vi "ROI entry-Previous ROI compat-FOV.vi"(8 "error in (no error)":errorcluster, 9 "Proceed":bool=TRUE, 11 "Old ROI file path":path) -> (0 "error out":errorcluster, 1 "Proceed":bool, 3 "Old ROI file path (dup)":path)   [LabVIEW 2017]
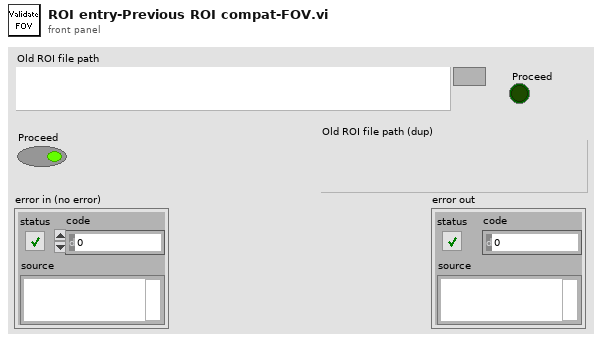
[diagram p1: front panel]
types:
  T1 = typedef "Fixed strings.ctl" = cluster{"ROI file name":string, "Normalised ROI file name":string, "Zplane Pockels values file name":string, "Functional data folder name":string, "Experiment Header file name":string, "Z-stack images folder name":string, "Groups setup rel. path":string, "Groups text file rel. path":string, "TDMS files folder name (F.img)":string, "TDMS files folder name (V.acq)":string, "TDMS files folder name (Pl.acq)":string, "Cycle rel times sequence file":string, "Dynamically called VIs folder name":string, "Time Series folder base name":string}
  T2 = typedef "AOL_Globals.ctl" = cluster{"Imaging Protocol":T3, "Number of POI":u16, "Number of Miniscans":u16, "Number of Trials":u16, "Number of Cycles ":u64, "# Averaged Frames":u16, "Laser power (%)":u8, "Pockels":dbl, "Acquisition Length (sec)":dbl, "Fill time (us)":dbl, "POI Dwell time (us)":dbl, "Miniscan Dwell time per pixel (us)":dbl, "PMT 1":dbl, "PMT 2":dbl, "Back Apperture":dbl, "Frame Size":T4, "Center Frequency":dbl, "Field of View (norm)":dbl, "DwellTime (us)":dbl, "Wavelength (nm)":dbl, "Zoom":dbl, "AOL Z":dbl, "AOL Mode":T5, "GridXY":dbl, "GridZ":dbl, "TriggerPeriod (sec)":dbl, "Number of Pixels in Miniscan":u16, "Experiment folder path":path, "X centre":dbl, "Y centre":dbl, "Angle (degrees)":dbl, "Plane Mode":T6, "Threshold":u16[], "Regenerate Chirps":bool, "Rectangle ROI length (pixels)":u16, "Rectangle ROI height (pixels)":u16, "AOD fill":u16, "StartupDelay":i32, "Samples Wait after Trigger":u16, "Slip Cycle":u32, "Add Cycle":bool, "Functional Mode":T7, "Z Start":dbl, "Z Stop":dbl, "# Planes":i32}
  T3 = typedef "Imaging Protocols enum.ctl" = enum16{"AOL Z-Stack", "Motor Z Stack", "Functional Acquisition", "Single Plane Acquisition", "Volume Acquisition", "Live Imaging", "Live Plane Imaging", "Live Volume Imaging"}
  T4 = typedef "Frame Size.ctl" = u16
  T5 = typedef "AOL modes.ctl" = enum16{"Raster", "Structural", "Pointing", "Mini Scan", "Alignment"}
  T6 = typedef "Plane Mode.ctl" = u16
  T7 = typedef "Functional Mode.ctl" = enum16{"Point", "Line", "Patch", "Plane", "Volume"}
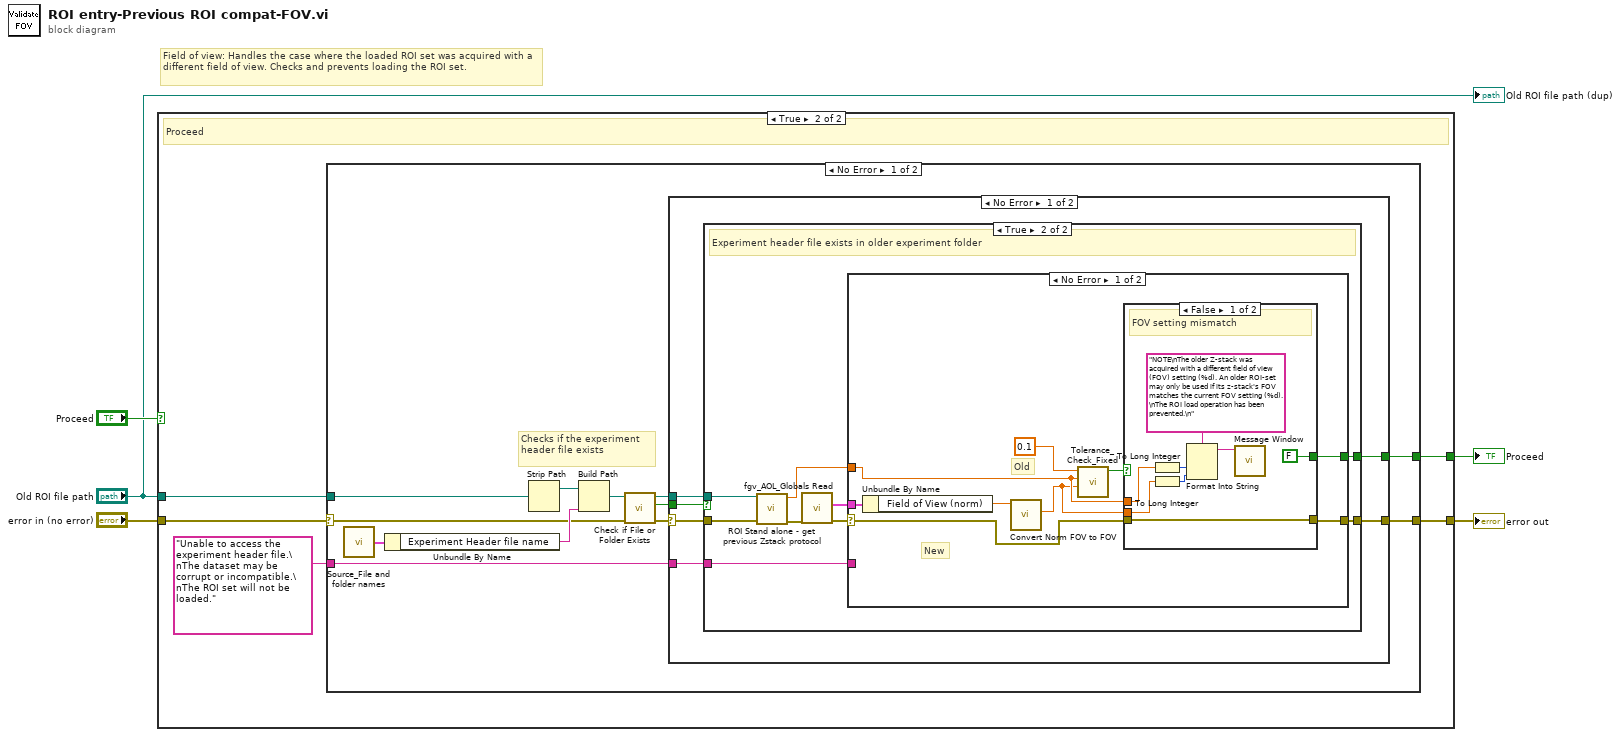
[diagram p0: block diagram]
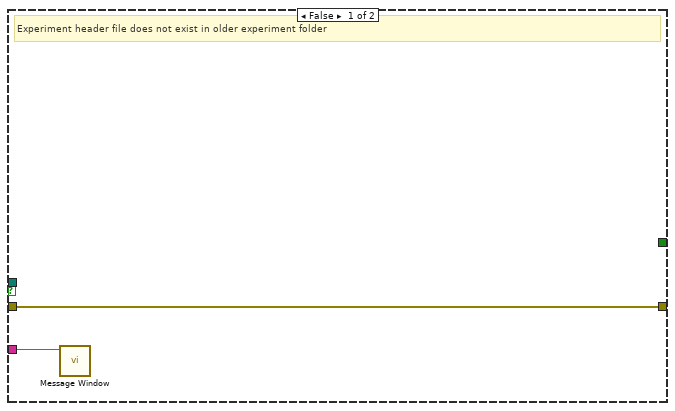
[diagram p3: hidden frame]
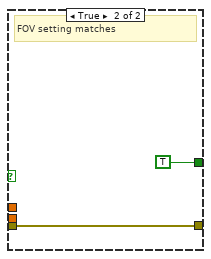
[diagram p4: hidden frame]
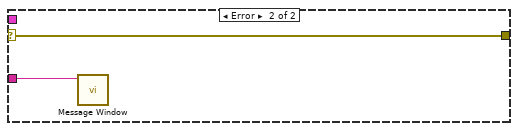
[diagram p5: hidden frame]
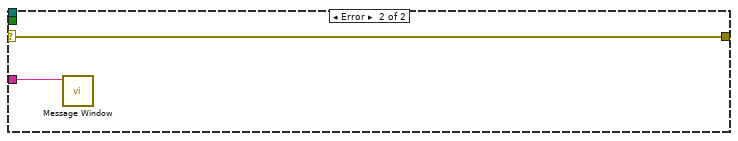
[diagram p6: hidden frame]
diagram:
  # "Field of view: Handles the case where the loaded ROI set was acquired with a different field of view. Checks and prevents loading the ROI set."
  n1 = case shown="True" "Proceed" {
    tunnel: "Old ROI file path" -> [_ w11]
    tunnel: [w6 w9] -> w5
    tunnel: "error in (no error)" -> [w6 w8]
    tunnel: [_ w7] -> w3
    frame False {
      # "Skip"
    }
    frame True {
      # "Proceed"
      n2 = case shown="No Error" w8 {
        selector: w8 -> [w14 w64]
        tunnel: w11 -> [w21 _]
        tunnel: [w17 _] -> w7
        tunnel: [w13 w64] -> w9
        tunnel: "Unable to access the experiment header file.\nThe dataset may be corrupt or incompatible.\nThe ROI set will not be loaded." ("Message string") -> [w12 _]
        frame No Error {
          # "Checks if the experiment header file exists"
          n3 = call "Source_File and folder names.vi"() -> ("Fixed strings"=w22:T1)  [unwired: 1 in]
          n4 = Unbundle By Name(w22) -> ("Experiment Header file name"=w19:string)
          n5 = Strip Path(path=w21) -> (stripped path=w20:path)  [unwired: 1 out]
          n6 = Build Path(base path=w20, name or relative path=w19) -> (appended path=w23:path)
          n7 = call <vilib>:"Check if File or Folder Exists.vi"("error in (no error)"=w14, "path"=w23) -> ("error out"=w15:errorcluster, "file or folder exists?"=w18:bool, "dup path"=w16:path)  [unwired: 7 in]
          n8 = case shown="No Error" w15 {
            selector: w15 -> [w26 w63]
            tunnel: w18 -> [w29 _]
            tunnel: [w28 _] -> w17
            tunnel: w16 -> [w27 _]
            tunnel: [w25 w63] -> w13
            tunnel: w12 -> [w24 w62]
            frame No Error {
              n9 = case shown="True" w29 {
                tunnel: [_ w39] -> w28
                tunnel: w27 -> [_ w34]
                tunnel: w26 -> [w31 w35]
                tunnel: [w31 w38] -> w25
                tunnel: w24 -> [w30 w36]
                frame False {
                  # "Experiment header file does not exist in older experiment folder"
                  n10 = call "Message Window.vi"("Message string"=w30) -> ()  [unwired: 10 in, 1 out]
                }
                frame True {
                  # "Experiment header file exists in older experiment folder"
                  n11 = call "ROI Stand alone - get previous Zstack protocol.vi"("error in (no error)"=w35, "path"=w34) -> ("error out"=w33:errorcluster, "field of view"=w32:dbl)  [unwired: 5 in, 3 out]
                  n12 = call "fgv_AOL_Globals Read.vi"("error in (no error)"=w33) -> ("error out"=w37:errorcluster, "AOL_Globals"=w40:T2)  [unwired: 8 in, 1 out]
                  n13 = case shown="No Error" w37 {
                    selector: w37 -> [w45 w61]
                    tunnel: w40 -> [w47 _]
                    tunnel: [w49 _] -> w39
                    tunnel: [w48 w61] -> w38
                    tunnel: w36 -> [_ w60]
                    tunnel: w32 -> [w42 _]
                    frame No Error {
                      # "New"
                      # "Old"
                      n14 = Unbundle By Name(w47) -> ("Field of View (norm)"=w46:dbl)
                      n15 = call "Convert Norm FOV to FOV.vi"("Field of View(norm)"=w46) -> ("FOV"=w41:dbl)  [unwired: 9 in, 1 out]
                      n16 = call <userlib>:"Tolerance_Check_Fixed.vi"("Value to check"=w41, "Setpoint"=w42, "Tolerance (+-)"=0.1) -> ("In Range"=w44:bool)  [unwired: 8 in]
                      n17 = case shown="False" w44 {
                        tunnel: [FALSE TRUE] -> w49
                        tunnel: w45 -> [w57 w58]
                        tunnel: [w57 w58] -> w48
                        tunnel: w42 -> [w51 _]
                        tunnel: w41 -> [w50 _]
                        frame False {
                          # "FOV setting mismatch"
                          n18 = To Long Integer(number=w51) -> (32bit integer=w55:i32)
                          n19 = To Long Integer(number=w50) -> (32bit integer=w52:i32)
                          n20 = Format Into String(format string="NOTE\nThe older Z-stack was acquired with a different field of view (FOV) setting (%d). An older ROI-set may only be used if its z-stack's FOV matches the current FOV setting (%d).\nThe ROI load operation has been prevented.\n" ("Message string"), w55, w52) -> (resulting string=w54:string)  [unwired: 2 in, 1 out]
                          n21 = call "Message Window.vi"("Message string"=w54) -> ()  [unwired: 10 in, 1 out]
                        }
                        frame True {
                          # "FOV setting matches"
                        }
                      }
                    }
                    frame Error {
                      n22 = call "Message Window.vi"("Message string"=w60) -> ()  [unwired: 10 in, 1 out]
                    }
                  }
                }
              }
            }
            frame Error {
              n23 = call "Message Window.vi"("Message string"=w62) -> ()  [unwired: 10 in, 1 out]
            }
          }
        }
        frame Error {
        }
      }
    }
  }
  "error out" <- w5
  "Proceed" <- w3
  "Old ROI file path (dup)" <- "Old ROI file path"
